vi "Read Tab Control.vi"(8 "error in":errorcluster, 11 "Tab Control in":refnum<vi>) -> (0 "error out":errorcluster, 1 "Value":string[](array[string]), 2 "Interpret As Unicode":bool, 3 "Tab Control out":refnum<vi>)   [LabVIEW 2020, in "G-Unicode.lvlib"]
uses:
  G-Unicode.lvlib
  Unicode/Controls/String Encoding.ctl
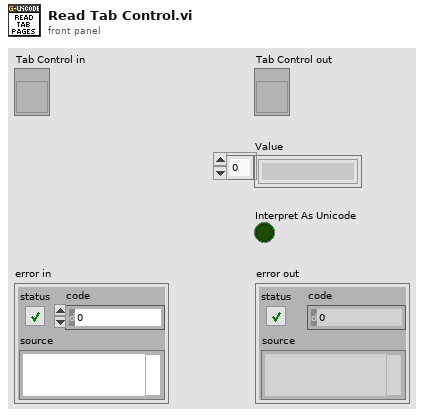
[diagram p1: front panel]
types:
  T1 = typedef "G-Unicode.lvlib/String Encoding.ctl" = enum16{"ANSI", "UTF-8", "UTF-16LE", "UTF-16BE", "Unknown"}
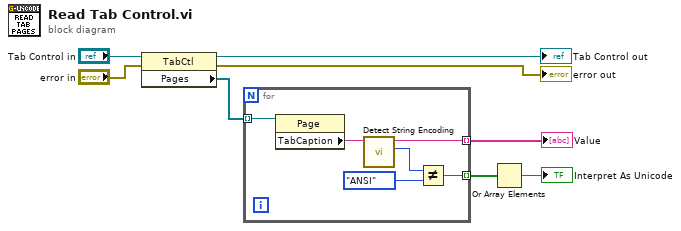
[diagram p0: block diagram]
diagram:
  n1 = property class="TabCtl"(reference="Tab Control in", error in="error in") -> (reference out=→"Tab Control out":refnum<vi>, error out=→"error out":errorcluster, "Pages"=w4:refnum<vi>[])
  n2 = for {
    tunnel: w4 -> [w14] mode=indexing
    tunnel: [w12] -> w3 mode=indexing
    tunnel: [w9] -> w1 mode=indexing
    n3 = property class="Page"(reference=w14) -> ("TabCaption"=w13:string)  [unwired: 1 in, 2 out]
    n4 = call "Detect String Encoding.vi"("String"=w13) -> ("Encoding"=w11:T1, "String out"=w12:string)  [unwired: 8 in, 1 out]
    n5 = Not Equal?(x=w11, y=String_Encoding."ANSI" ("Encoding")) -> (x != y?=w9:bool)
  }
  "Value" <- w3
  n6 = Or Array Elements(Boolean array=w1) -> (logical OR=→"Interpret As Unicode":bool)
